vi "Path To Unix Path.vi"(0 "path":path) -> (2 "unix path":string)   [LabVIEW 2013, in "libssh2_integration_tests.lvlib" / "Server Fixture.lvclass"]
doc: "Convert path to unix path."
uses:
  Server Fixture.lvclass
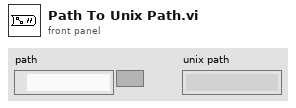
[diagram p1: front panel]
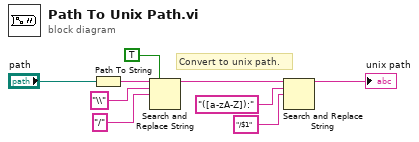
[diagram p0: block diagram]
diagram:
  # "Convert to unix path."
  n1 = Path To String(path="path") -> (string=w9:string)
  n2 = Search and Replace String(replace all?=TRUE ("replace all? (F)"), input string=w9, search string="\\", replace string="/" ("replace string (\"\")")) -> (result string=w5:string)  [unwired: 4 in, 3 out]
  n3 = Search and Replace String(input string=w5, search string="([a-zA-Z]):", replace string="/$1" ("replace string (\"\")")) -> (result string=→"unix path":string)  [unwired: 5 in, 3 out]
